vi "Log Data.vi"(4 "Volatge Y":dbl[](array[numeric]), 5 "Ending edges":i32[](array[numeric]), 6 "Starting edges":i32[](array[numeric]), 7 "Last request":bool, 8 "error in (no error)":errorcluster, 9 "Volatge X":dbl[](array[numeric]), 10 "Frequency":dbl[](array[numeric]), 11 "Spectrum Recorder in":refnum<class "Spectrum Recorder too.lvclass">) -> (0 "error out":errorcluster, 2 "Result":refnum<class "Acquired Result.lvclass">, 3 "Spectrum Recorder out":refnum<class "Spectrum Recorder too.lvclass">)   [LabVIEW 2016, in "Spectrum Recorder too.lvclass"]
uses:
  Spectrum Recorder too.lvclass
  C:/github/LabActor/Worker/Worker.lvclass
  NHMFL_Core/Libraries/Instruments/Results/Acquired Result/Acquired Result.lvclass
  Worker/Worker.lvclass/Worker.ctl
  Spectrum Recorder too.lvclass/Spectrum Recorder too.ctl
  NHMFL_Core/Libraries/Instruments/Results/Acquired Result/Acquired Result.lvclass/Acquired Result.ctl
  Worker/Read Cycle count.vi
  NHMFL_Core/Libraries/Instruments/Results/Acquired Result/Write Cycle count.vi
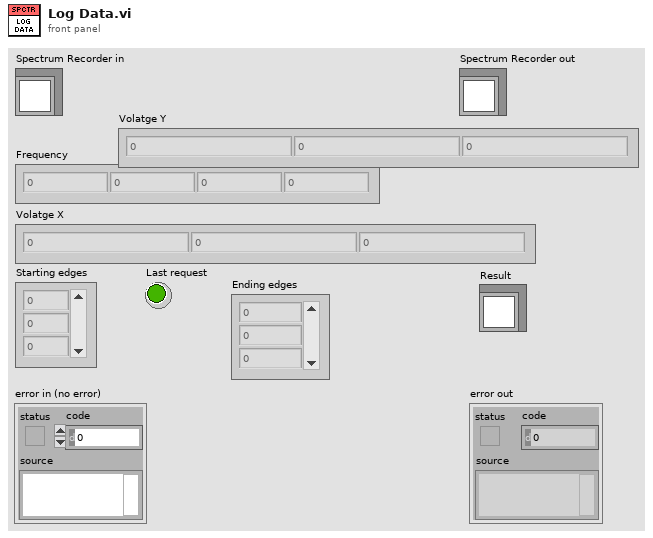
[diagram p1: front panel]
types:
  T1 = typedef "Stream Segment.ctl" = cluster{"Start":i32, "End":i32, "Open":bool, "Close":bool}
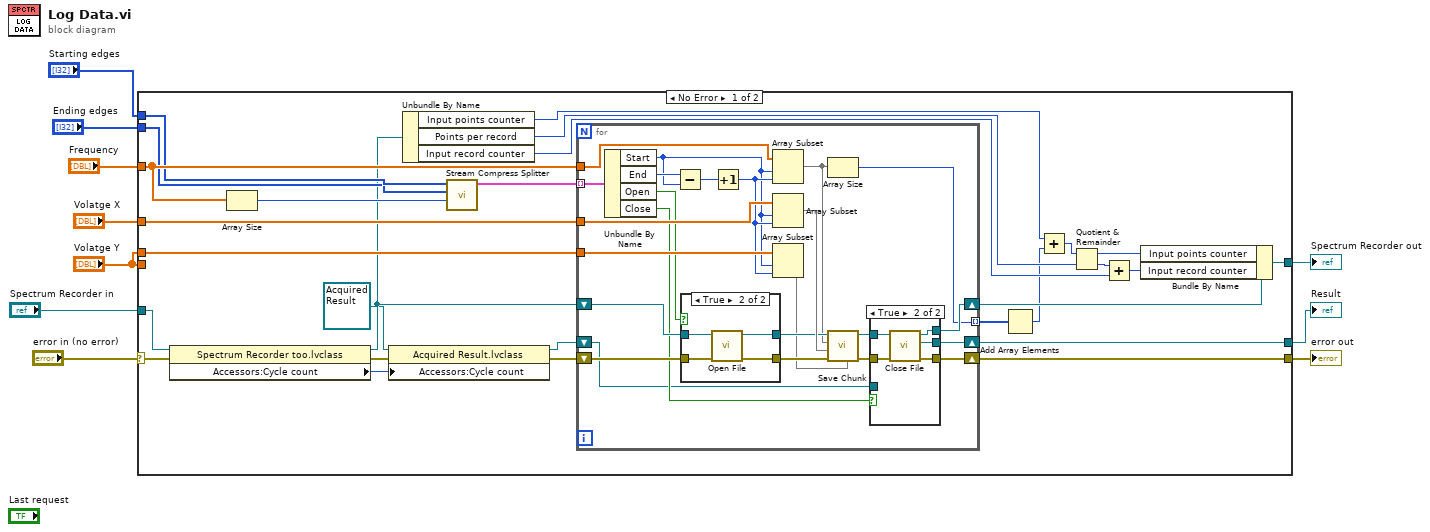
[diagram p0: block diagram]
diagram:
  n1 = case shown="No Error" "error in (no error)" {
    selector: "error in (no error)" -> [w34 w78]
    tunnel: [w37 w78] -> w9
    tunnel: [w26 w77] -> w7
    tunnel: "Spectrum Recorder in" -> [w16 w77]
    tunnel: "Starting edges" -> [w24 _]
    tunnel: "Volatge X" -> [w35 _]
    tunnel: "Frequency" -> [w36 _]
    tunnel: "Ending edges" -> [w23 _]
    tunnel: "Volatge Y" -> [_ _]
    tunnel: "Volatge Y" -> [w25 _]
    tunnel: [w18 _] -> w1
    frame No Error {
      n2 = property class="Spectrum Recorder too.lvclass"(reference=w16, error in=w34) -> (reference out=w15:refnum<class "Spectrum Recorder too.lvclass">, error out=w17:errorcluster, "Accessors:Cycle count"=w11:i32)
      n3 = Array Size(array=w36) -> (size(s)=w22:i32)
      n4 = property class="Acquired Result.lvclass"(reference=refnum<class "Acquired Result.lvclass"> refnum ("Acquired Result.lvclass"), error in=w17, "Accessors:Cycle count"=w11) -> (reference out=w12:refnum<class "Acquired Result.lvclass">, error out=w14:errorcluster)
      n5 = Unbundle By Name(w15) -> ("Input points counter"=w33:i32, "Points per record"=w31:i32, "Input record counter"=w29:i32)
      n6 = call "Stream Compress Splitter.vi"("Array lengh"=w22, "Ending edges"=w23, "Starting edges"=w24) -> ("Segments"=w21:T1[])  [unwired: 8 in]
      n7 = for {
        shift-right: [w46] -> w37
        shift-left: w14 -> [w60]
        tunnel: w36 -> [w62]
        tunnel: w35 -> [w61]
        shift-right: [w47] -> w38
        shift-left: w15 -> [w57]
        tunnel: w25 -> [w54]
        tunnel: w21 -> [w52] mode=indexing
        tunnel: [w43] -> w20 mode=indexing
        shift-right: [w42] -> w18
        shift-left: w12 -> [w41]
        n8 = Unbundle By Name(w52) -> ("Start"=w39:i32, "End"=w40:i32, "Open"=w49:bool, "Close"=w44:bool)
        n9 = Subtract(x=w40, y=w39) -> (x-y=w51:i32)
        n10 = case shown="True" w49 {
          tunnel: w60 -> [w71 w76]
          tunnel: [w71 w75] -> w58
          tunnel: w57 -> [w72 w74]
          tunnel: [w72 w73] -> w56
          frame False {
          }
          frame True {
            n11 = call-dynamic "Open File.vi"("error in (no error)"=w76, "Spectrum Recorder in"=w74) -> ("error out"=w75:errorcluster, "Spectrum Recorder out"=w73:refnum<class "Spectrum Recorder too.lvclass">)  [unwired: 8 in]
          }
        }
        n12 = Increment(x=w51) -> (x+1=w50:i32)
        n13 = Array Subset(array=w62, index=w39, length=w50) -> (w55:dbl[])
        n14 = Array Subset(array=w61, index=w39, length=w50) -> (w59:dbl[])
        n15 = Array Subset(array=w54, index=w39, length=w50) -> (w53:dbl[])
        n16 = Array Size(array=w55) -> (size(s)=w43:i32)
        n17 = call-dynamic "Save Chunk.vi"("Volatge Y"=w53, "error in (no error)"=w58, "Voltage X"=w59, "Frequency"=w55, "Spectrum Recorder in"=w56) -> ("error out"=w45:errorcluster, "Spectrum Recorder out"=w48:refnum<class "Spectrum Recorder too.lvclass">)  [unwired: 5 in]
        n18 = case shown="True" w44 {
          tunnel: w48 -> [w65 w70]
          tunnel: [w65 w69] -> w47
          tunnel: [w64 w68] -> w46
          tunnel: w45 -> [w64 w67]
          tunnel: [w63 w66] -> w42
          tunnel: w41 -> [w63 _]
          frame False {
          }
          frame True {
            n19 = call-dynamic "Close File.vi"("error in (no error)"=w67, "Spectrum Recorder in"=w70) -> ("error out"=w68:errorcluster, "Acquired Result.lvclass"=w66:refnum<class "Acquired Result.lvclass">, "Spectrum Recorder out"=w69:refnum<class "Spectrum Recorder too.lvclass">)  [unwired: 7 in]
          }
        }
      }
      n20 = Add Array Elements(numeric array=w20) -> (sum=w19:i32)
      n21 = Add(x=w33, y=w19) -> (x+y=w32:i32)
      n22 = Quotient & Remainder(x=w32, y=w31) -> (x-y*floor(x/y)=w30:i32, floor(x/y)=w28:i32)
      n23 = Add(x=w28, y=w29) -> (x+y=w27:i32)
      n24 = Bundle By Name(cluster=w38, "Input points counter"=w30, "Input record counter"=w27) -> (w26:refnum<class "Spectrum Recorder too.lvclass">)
    }
    frame Error {
    }
  }
  "error out" <- w9
  "Spectrum Recorder out" <- w7
  "Result" <- w1
